vi "Test Process Asynchronous Action Stopped when Process Stopped.vi"(8 "error in (no error)":errorcluster, 11 "Helper Loop Test In":refnum<class "Process Test.lvclass">) -> (0 "error out":errorcluster, 3 "Helper Loop Test Out":refnum<class "Process Test.lvclass">)   [LabVIEW 2020, in "Process Test.lvclass"]
uses:
  Process Test.lvclass
  C:/Program Files (x86)/National Instruments/LabVIEW 2020/vi.lib/Astemes/LUnit/Test Case.lvclass
  Framework/Async Handler/Async Handler.lvclass
  Framework/Process/Process.lvclass/Process.ctl
  <vilib>/Astemes/LUnit/Test Case.lvclass/Test Case.ctl
  <vilib>/Astemes/LUnit/LUnit Assertion Result.lvclass/LUnit Assertion Result.ctl
  <vilib>/Astemes/LUnit/LUnit Test Case Result.lvclass/LUnit Test Case Result.ctl
  <vilib>/Astemes/LUnit/LUnit Method Result.lvclass/LUnit Method Result.ctl
  ff6210df-d80d-4043-ac84-bb28d4723d35.vi
  27698d7c-1d27-4f20-94d5-aa7beea38d40.vi
  3c03c699-6819-427c-a8c0-7eedb7611303.vi
  Framework/Process/Public/Lifecycle/Get Lifecycle State.vi
  Framework/Broadcast Event Helpers/Dequeue Broadcast Message by Message Cluster.vi
  <vilib>/Astemes/LUnit/Palette/Pass.vi
  <vilib>/Astemes/LUnit/Palette/Fail.vi
  <vilib>/Astemes/LUnit/Compare Variants.vi
  <vilib>/Astemes/LUnit/Describe Comparison.vi
  <vilib>/Astemes/LUnit/Set Assertion Type.vi
  Framework/Process/Private/SubVIs/Wait for finish.vi
  Framework/Process/Protected/Messaging/Enqueue Message.vi
  Framework/Process/Private/SubVIs/Set Lifecycle State.vi
  <vilib>/Astemes/LUnit/Add test result.vi
  <vilib>/Astemes/LUnit/LUnit Write Message.vi
  <vilib>/Astemes/LUnit/LUnit Write Description.vi
  <vilib>/Astemes/LUnit/LUnit Write Skipped.vi
  <vilib>/Utility/error.llb/Clear Errors.vi
  Framework/Broadcast Event Helpers/Execution timer.vi
  <vilib>/Astemes/LUnit/LUnit Write Passed.vi
  <vilib>/Astemes/LUnit/Variant to string.vi
  <vilib>/Astemes/LUnit/LUnit Write Assertion Type.vi
  Framework/Process/Private/SubVIs/Handle Debug Data.vi
  <vilib>/Astemes/LUnit/LUnit Record Assertion Result.vi
  Framework/Logging/Log Debug.vi
  <vilib>/AdvancedString/1D String Array to Delimited String.vi
  <vilib>/Utility/High Resolution Relative Seconds.vi
  <vilib>/Astemes/LUnit/LUnit Aggregate Assertion Results.vi
  <vilib>/Astemes/LUnit/Assertion Result/LUnit Read Status.vi
  <vilib>/Astemes/LUnit/LUnit Read Message.vi
  <vilib>/Astemes/LUnit/LUnit Read Description.vi
  <vilib>/Astemes/LUnit/Method Result/LUnit Merge Status.vi
  <vilib>/Astemes/LUnit/LUnit Concatenate result strings.vi
  <vilib>/Utility/error.llb/Error Cluster From Error Code.vi
  Framework/Broadcast Event Helpers/Dequeue Broadcast Message.vi
  <vilib>/Utility/Data Type/Get Type Information.vi
  <vilib>/Utility/LVClass/Get LV Class Name.vi
  Framework/Process/Public/Read Name.vi
  <vilib>/Astemes/LUnit/LUnit Assertion Result.lvclass
  Framework/Process/Process.lvclass
  Process Test.lvclass/Process Test.ctl
  <vilib>/Astemes/LUnit/Test Case.lvclass
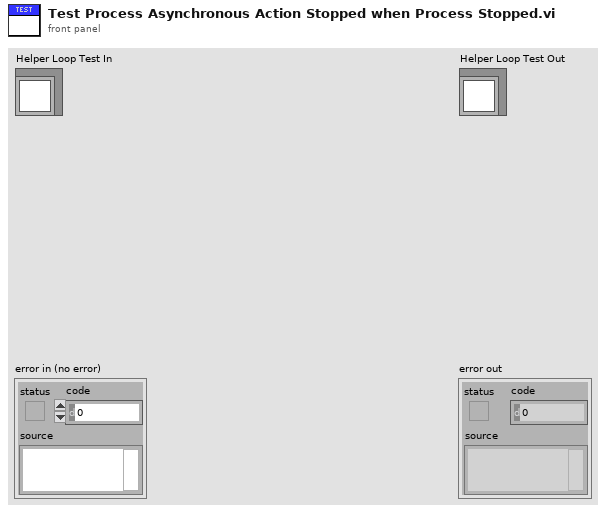
[diagram p1: front panel]
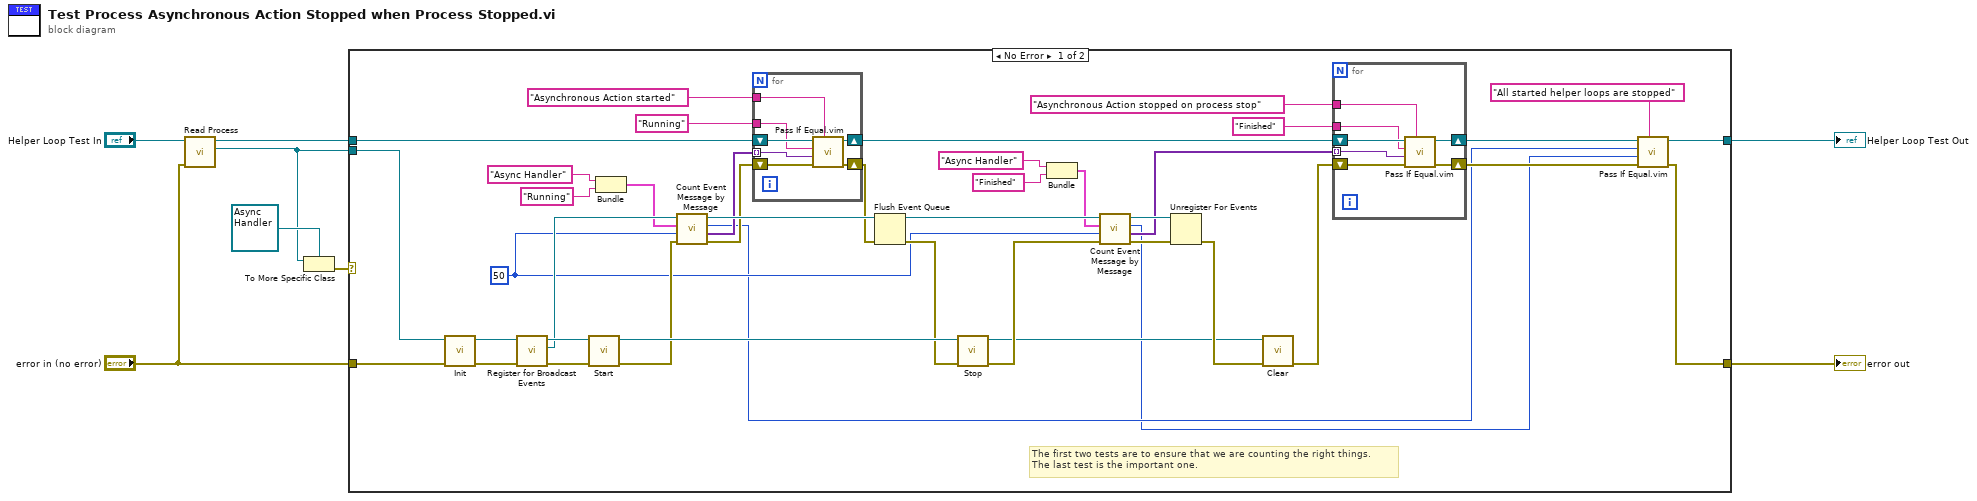
[diagram p0: block diagram]
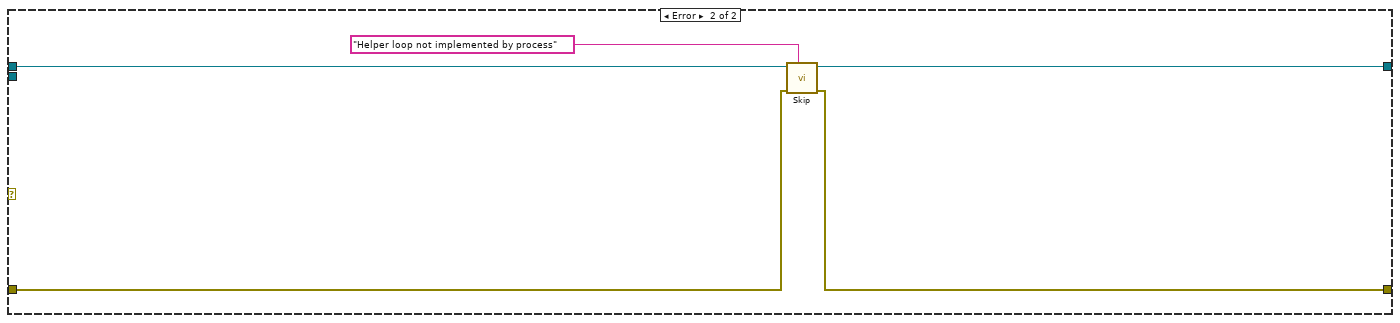
[diagram p2: hidden frame]
diagram:
  n1 = call "Read Process.vi"("error in (no error)"="error in (no error)", "Process Test in"="Helper Loop Test In") -> ("Process.lvclass"=w1:refnum<class "Process.lvclass">, "Process Test out"=w5:refnum<class "Process Test.lvclass">)  [unwired: 7 in, 1 out]
  n2 = To More Specific Class(target class=refnum<class "Async Handler.lvclass"> refnum ("Asynchronous Action.lvclass"), reference=w1) -> (error out=w3:errorcluster)  [unwired: 1 in, 1 out]
  n3 = case shown="No Error" w3 {
    tunnel: [w21 w68] -> w8
    tunnel: "error in (no error)" -> [w44 w67]
    tunnel: [w19 w66] -> w7
    tunnel: w5 -> [w31 w69]
    tunnel: w1 -> [w36 _]
    frame No Error {
      w30 = 50 ("Timeout (-1)")
      # "The first two tests are to ensure that we are counting the right things. \nThe last test is the important one."
      n4 = call-dynamic "Init.vi"("error in (no error)"=w44, "Process In"=w36) -> ("error out"=w49:errorcluster, "Process Out"=w50:refnum<class "Process.lvclass">)  [unwired: 8 in]
      n5 = call "Register for Broadcast Events.vi"("error in (no error)"=w49, "Process In"=w50) -> ("error out"=w47:errorcluster, "Event Registration Refnum Out"=w35:refnum<event-registration>, "Process Out"=w48:refnum<class "Process.lvclass">)  [unwired: 7 in]
      n6 = call "Start.vi"("error in (no error)"=w47, "Process In"=w48) -> ("error out"=w33:errorcluster, "Process Out"=w46:refnum<class "Process.lvclass">)  [unwired: 7 in, 1 out]
      n7 = Bundle("y"="Async Handler", "Description"="Running") -> (w12:cluster{"y":string, "Description":string})  [unwired: 1 in]
      n8 = call "Count Event Message by Message.vi"("error in (no error)"=w33, "Timeout"=w30, "Message"=w12, "Event Registration Refnum in"=w35) -> ("error out"=w29:errorcluster, "Message Data"=w25:variant[], "Count"=w18:i32, "Event Registration Refnum out"=w34:refnum<event-registration>)  [unwired: 4 in]
      n9 = for {
        tunnel: "Asynchronous Action started" ("Description") -> [w53]
        tunnel: "Running" ("Description") -> [w52]
        shift-right: [w57] -> w32
        shift-left: w31 -> [w56]
        shift-right: [w54] -> w28
        shift-left: w29 -> [w55]
        tunnel: w25 -> [w51] mode=indexing
        n10 = call "Pass If Equal.vim"("Description"=w53, "error in (no error)"=w55, "Actual"=w51, "Expected"=w52, "LUnit Test Case In"=w56) -> ("error out"=w54:errorcluster, "LUnit Test Case Out"=w57:refnum<class "Process Test.lvclass">)  [unwired: 5 in]
      }
      n11 = Flush Event Queue(0:w34, 3:w28) -> (8:w41:refnum<event-registration>, 11:w40:errorcluster)  [unwired: 4 in, 1 out]
      n12 = call "Stop.vi"("error in (no error)"=w40, "Process In"=w46) -> ("error out"=w39:errorcluster, "Process Out"=w38:refnum<class "Process.lvclass">)  [unwired: 7 in, 1 out]
      n13 = Bundle("y"="Async Handler", "Description"="Finished") -> (w9:cluster{"y":string, "Description":string})  [unwired: 1 in]
      n14 = call "Count Event Message by Message.vi"("error in (no error)"=w39, "Timeout"=w30, "Message"=w9, "Event Registration Refnum in"=w41) -> ("error out"=w37:errorcluster, "Message Data"=w24:variant[], "Count"=w17:i32, "Event Registration Refnum out"=w43:refnum<event-registration>)  [unwired: 4 in]
      n15 = Unregister For Events(event registration refnum=w43, error in=w37) -> (error out=w42:errorcluster)
      n16 = call-dynamic "Clear.vi"("error in (no error)"=w42, "Process In"=w38) -> ("error out"=w45:errorcluster)  [unwired: 9 in]
      n17 = for {
        tunnel: w24 -> [w61] mode=indexing
        shift-right: [w62] -> w20
        shift-left: w45 -> [w64]
        shift-right: [w63] -> w22
        shift-left: w32 -> [w60]
        tunnel: "Asynchronous Action stopped on process stop" ("Description") -> [w59]
        tunnel: "Finished" ("Description") -> [w58]
        n18 = call "Pass If Equal.vim"("Description"=w59, "error in (no error)"=w64, "Actual"=w61, "Expected"=w58, "LUnit Test Case In"=w60) -> ("error out"=w62:errorcluster, "LUnit Test Case Out"=w63:refnum<class "Process Test.lvclass">)  [unwired: 5 in]
      }
      n19 = call "Pass If Equal.vim"("Description"="All started helper loops are stopped", "error in (no error)"=w20, "Actual"=w17, "Expected"=w18, "LUnit Test Case In"=w22) -> ("error out"=w19:errorcluster, "LUnit Test Case Out"=w21:refnum<class "Process Test.lvclass">)  [unwired: 5 in]
    }
    frame Error {
      n20 = call <vilib>:"Skip.vi"("Description"="Helper loop not implemented by process", "error in (no error)"=w67, "LUnit Test Case In"=w69) -> ("error out"=w66:errorcluster, "LUnit Test Case Out"=w68:refnum<class "Process Test.lvclass">)  [unwired: 7 in]
    }
  }
  "error out" <- w7
  "Helper Loop Test Out" <- w8
